vi "fpga_all_example2.vi"() -> ()   [LabVIEW 2020]
uses:
  controls/enum.ctl
  <vilib>/Platform/TimedLoop/XDataNode/timing_clust.ctl
  <vilib>/Platform/TimedLoop/XDataNode/nitl_modes.ctl
  <vilib>/Platform/TimedLoop/XDataNode/wakeup.ctl
  <vilib>/rvi/Emulation/niFpgaGetClockAttributes.vi
  <vilib>/rvi/Emulation/niFpgaSctlEmulationGetInTimedLoop.vi
  <vilib>/rvi/Emulation/niFpgaEmulationReportErrorSimple.vi
  <vilib>/rvi/Emulation/niFpgaCriticalErrorInLSC.vi
  <vilib>/rvi/Emulation/niFpgaProcessEmulError.vi
  <vilib>/rvi/eio/common/nirviEmuTemplateMethod_errors.vi
  lib/Cast-EPICS/cast u64 to u-64-64.vi
  lib/Cast-EPICS/cast u-64-64 to u64.vi
  lib/Cast-EPICS/cast u64 to u-64-0.vi
  lib/Cast-EPICS/cast u-64-0 to u64.vi
  lib/Cast-EPICS/cast u64 to u-64-32.vi
  lib/Cast-EPICS/cast u-64-32 to u64.vi
  lib/Cast-EPICS/cast u64 to s-64-0.vi
  lib/Cast-EPICS/cast s-64-0 to u64.vi
  lib/Cast-EPICS/cast u64 to s-64-64.vi
  lib/Cast-EPICS/cast s-64-64 to u64.vi
  lib/Cast-EPICS/cast u64 to s-64-32.vi
  lib/Cast-EPICS/cast s-64-32 to u64.vi
  <vilib>/Platform/TimedLoop/XDataNode/XDataNode.xnode
  <vilib>/eio/EIONode/EIONode.xnode
  <vilib>/Platform/TimedLoop/XDataNode/XDNodeRunTimeDep.lvlib
  lib/Scaler-EPICS/scaler.lvlib
  lib/Cast-EPICS/fixedpoint-cast.lvlib
panel:
  out "MBBI0":T1
  out "MBBI1":T1
  in  "MBBO1":T1
  in  "MBBO0":T1
  out "AI3":sgl format="%.2f"
  out "AI2":sgl format="%.2f"
  out "AI1":sgl format="%.2f"
  out "AI0":sgl format="%.2f"
  in  "AO3":sgl
  in  "AO2":sgl
  in  "AO1":sgl
  in  "AO0":sgl
  out "fixedpoint_i 1":fxp<+,64,64> format="%.20f"
  out "FXP1":u64
  out "fixedpoint_i 2":fxp<+,64,0> format="%#_20g"
  out "FXP2":u64
  out "fixedpoint_i 3":fxp<+,64,32> format="%#_20g"
  out "FXP3":u64
  out "fixedpoint_i 4":fxp<+/-,64,0> format="%#_20g"
  out "FXP4":u64
  out "fixedpoint_i 5":fxp<+/-,64,64> format="%.20f"
  out "FXP5":u64
  out "fixedpoint_i 6":fxp<+/-,64,32> format="%#_20g"
  out "FXP6":u64
  in  "FXP1":u64
  in  "FXP2":u64
  in  "FXP3":u64
  in  "FXP4":u64
  in  "FXP5":u64
  in  "FXP6":u64
  out "AnalogInputs_Scaler":fxp<+/-,20,5>[](array[numeric]) format="%.17g"
  out "Looptime":u32
  in  "Enable_SCALER":bool
  in  "OneShot_SCALER":bool
  in  "SampleAnalog_SCALER":bool
  in  "Gate_SCALER":bool[](array[boolean])=[FALSE, FALSE, FALSE, FALSE, FALSE]
  in  "PresetValues_SCALER":u32[](array[numeric])=[0, 0, 0, 0, 0]
  in  "fxp_ShiftLeft_SCALER":u64
  out "Done_SCALER":bool
  out "fxp_AnalogOutput0_SCALER":u64
  out "fxp_AnalogOutput1_SCALER":u64
  out "fxp_AnalogOutput2_SCALER":u64
  out "fxp_AnalogOutput3_SCALER":u64
  out "Counter_SCALER":u32[](array[numeric])
  out "BI_VECTOR":u64
  in  "BO3":bool
  out "BI_led3":bool
  out "BI_led2":bool
  in  "BO2":bool
  in  "BO1":bool
  out "BI_led1":bool
  out "BI_led0":bool
  in  "BO0":bool
  # "MBBI/MBBO Tests"
  # "BI/BO tests"
  # "AI/AO Tests"
  # "Scaler test"
  # "FXP test"
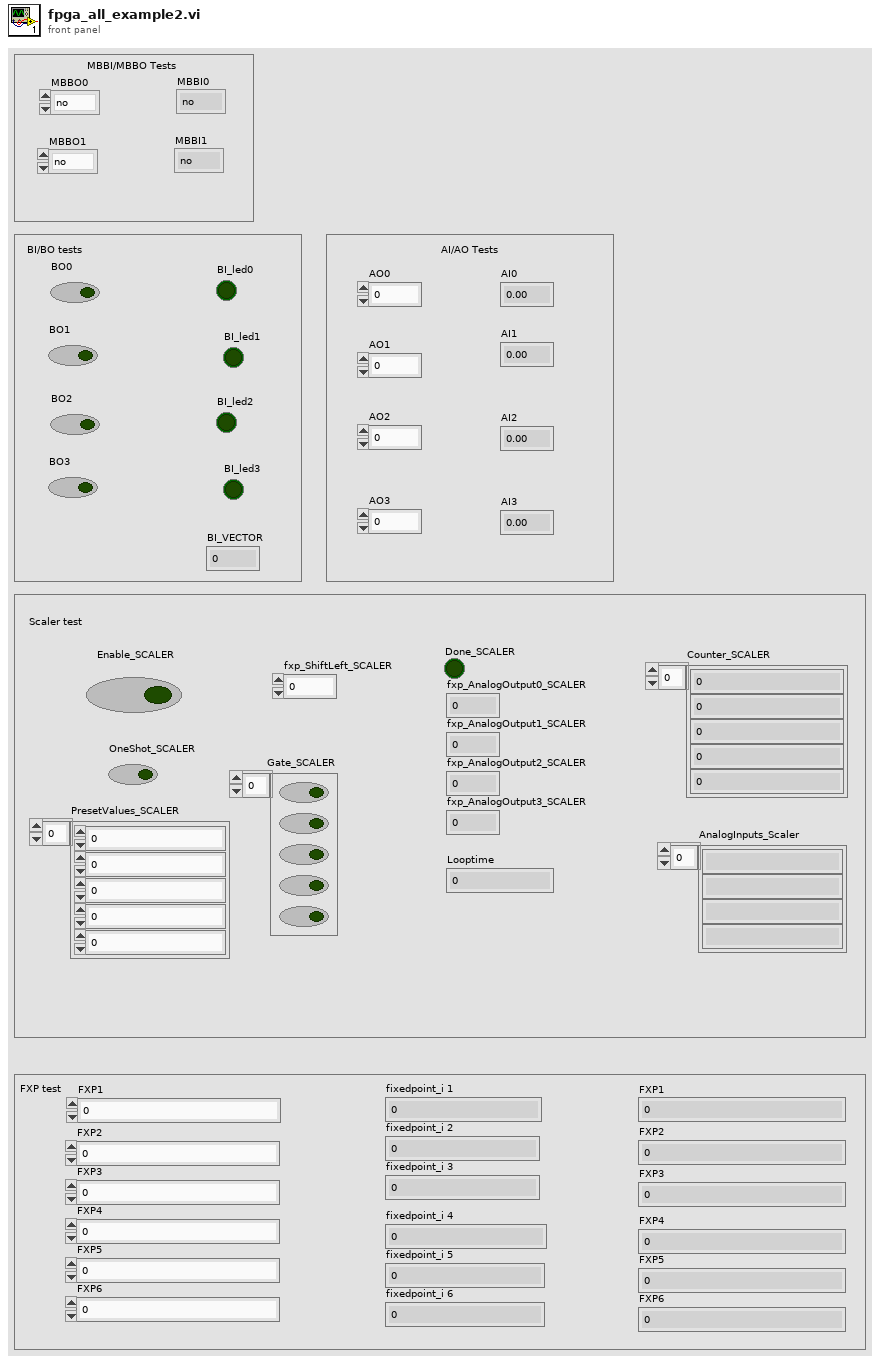
[diagram p1: front panel]
types:
  T1 = typedef "enum.ctl" = enum16{"no", "yes", "dont know"}
  T2 = typedef "XDNodeRunTimeDep.lvlib/timing_clust.ctl" = cluster{"Expected End [f-1]":u64, "Actual End [f-1]":u64, "Finished Late? [f-1]":bool, "Expected End [i-1]":u64, "Actual End [i-1]":u64, "Finished Late? [i-1]":bool, "Expected Start [i]":u64, "Actual Start [i]":u64, "Expected Start [f]":u64, "Actual Start [f]":u64, "Source Name":string, "Structure Name":string, "Period":i64, "Deadline":i64, "Offset":i64, "Start":i64, "Priority":i32, "Timeout":i32, "Mode":T3, "Wakeup Reason":T4, "Error":errorcluster, "Source Type":string, "Secondary Source Type":string, "Global End Time":u64, "Global Start Time":u64, "Frame Duration":u64, "Iteration Duration":u64, "Assigned CPU":i32, "I/O Scan Engine Mode":u32}
  T3 = typedef "XDNodeRunTimeDep.lvlib/nitl_modes.ctl" = enum32{"No Change", "Process missed periods, maintain original phase", "Discard missed periods, maintain original phase", "Process missed periods, ignore original phase", "Discard missed periods, ignore original phase"}
  T4 = typedef "XDNodeRunTimeDep.lvlib/wakeup.ctl" = enum32{"Normal", "Aborted", "Asynchronous wakeup", "Timing source error", "Timed loop error", "Timeout"}
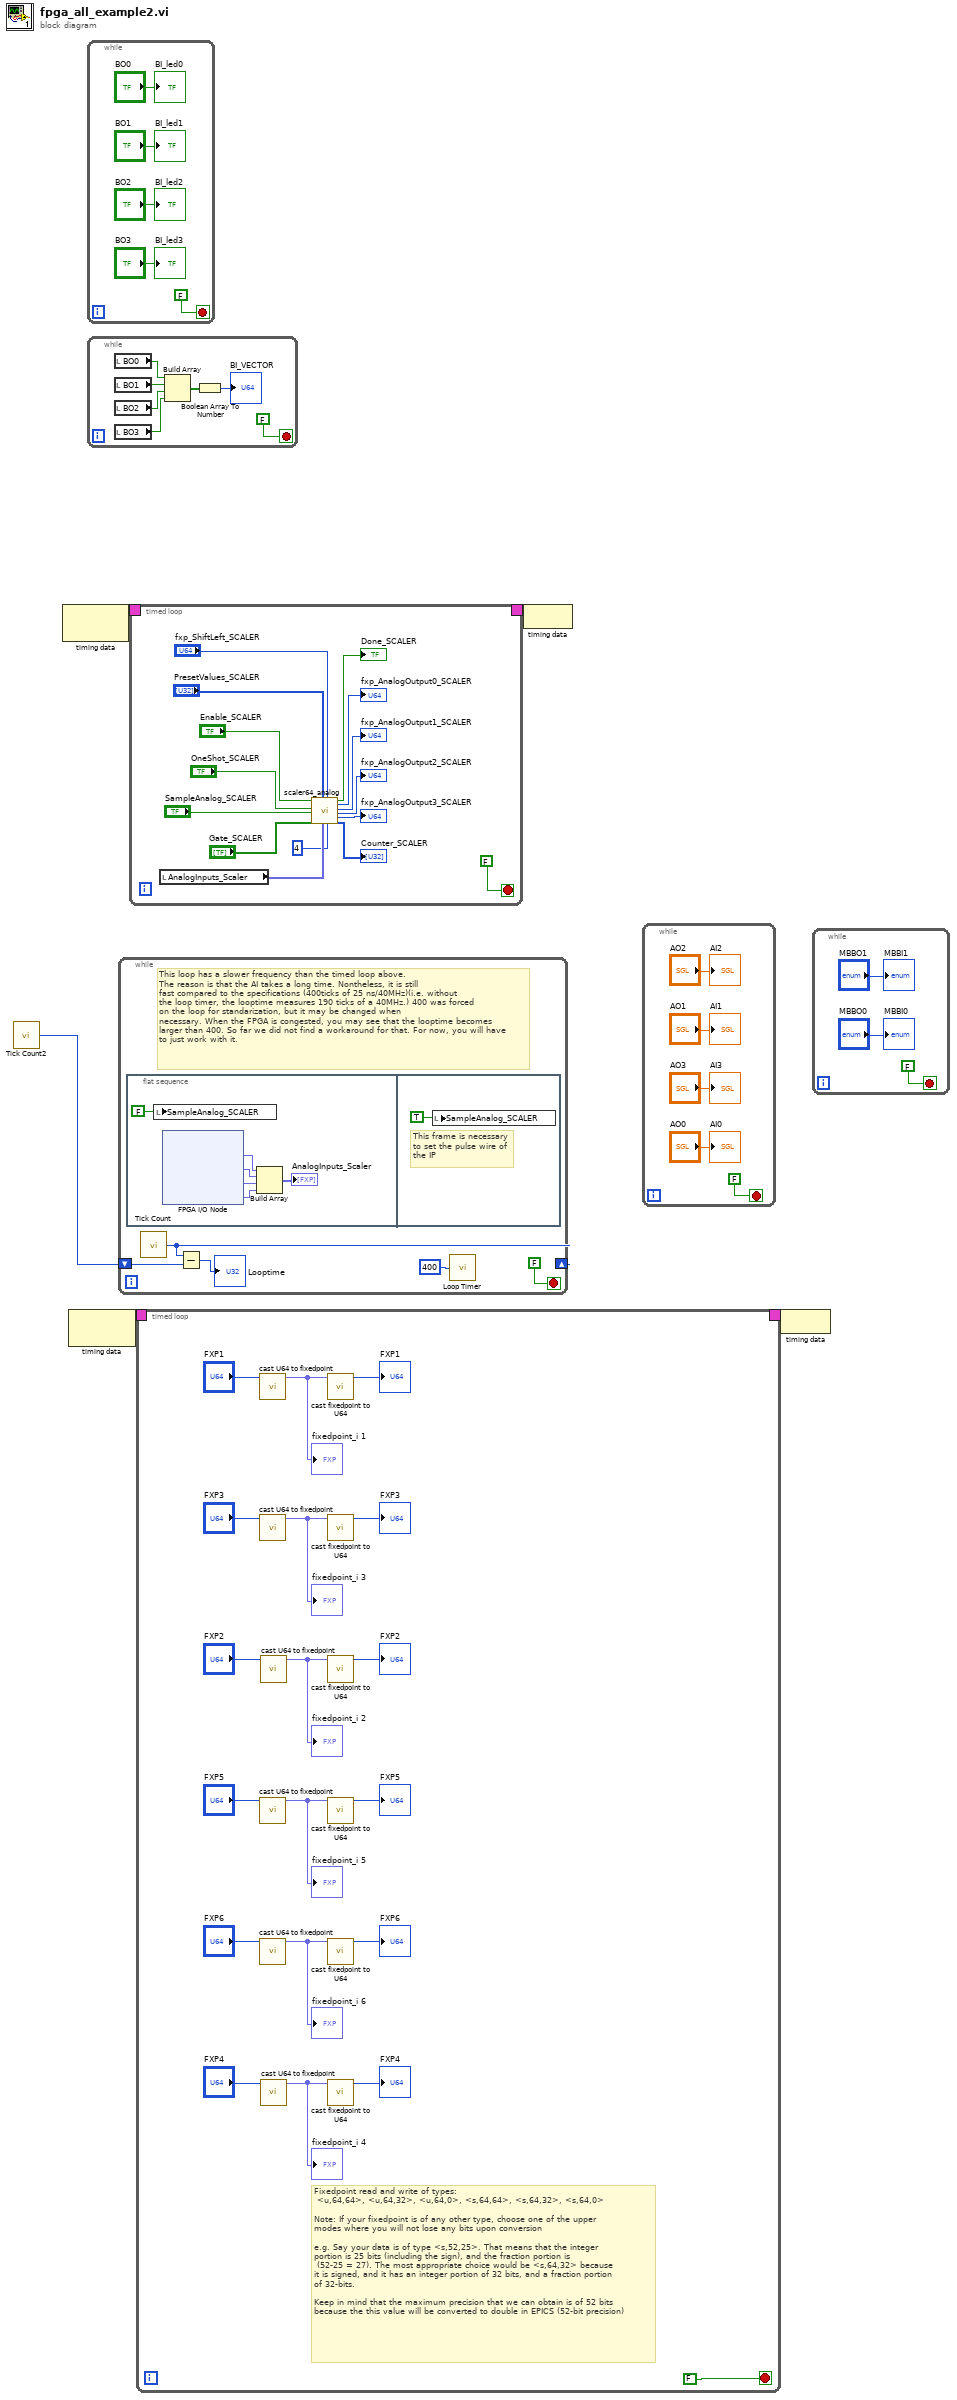
[diagram p0: block diagram]
diagram:
  n1 = call "Tick Count2"() -> ("Tick Count(Ticks)"=w3:u32)
  n2 = node-c288() -> (w5:T2)  [unwired: 1 in]
  n3 = node-c288() -> (w2:T2)  [unwired: 1 in]
  n4 = while {
    stop <- FALSE stop-if-true
    "BI_led0" <- "BO0"
    "BI_led1" <- "BO1"
    "BI_led2" <- "BO2"
    "BI_led3" <- "BO3"
  }
  n5 = while {
    stop <- FALSE stop-if-true
    n6 = local read "BO0"() -> (w14:bool)
    n7 = local read "BO1"() -> (w12:bool)
    n8 = local read "BO2"() -> (w13:bool)
    n9 = local read "BO3"() -> (w15:bool)
    n10 = Build Array(w14, w12, w13, w15) -> (w16:bool[])
    n11 = Boolean Array To Number(Boolean array=w16) -> (number=→"BI_VECTOR":u8)
  }
  n12 = while {
    shift-right: [w19] -> _
    shift-left: w3 -> [w20]
    stop <- FALSE stop-if-true
    # "This loop has a slower frequency than the timed loop above.\nThe reason is that the AI takes a long time. Nontheless, it is still\nfast compared to the specifications (400ticks of 25 ns/40MHz)(i.e. without \nthe loop timer, the looptime measures 190 ticks of a 40MHz.) 400 was forced \non the loop for standarization, but it may be changed when \nnecessary. When the FPGA is congested, you may see that the looptime becomes \nlarger than 400. So far we did not find a workaround for that. For now, you will have\nto just work with it."
    n13 = flat-sequence {
      frame #0 {
        n14 = local write "SampleAnalog_SCALER"(FALSE) -> ()
        n15 = xnode "FPGA I/O Node"() -> ("Mod4/AI0"=w28:fxp<+/-,20,5>, "Mod4/AI1"=w26:fxp<+/-,20,5>, "Mod4/AI2"=w25:fxp<+/-,20,5>, "Mod4/AI3"=w24:fxp<+/-,20,5>)  [unwired: 4 in, 4 out]
        n16 = Build Array(w28, w26, w25, w24) -> (→"AnalogInputs_Scaler":fxp<+/-,20,5>[])
      }
      frame #1 {
        # "This frame is necessary to set the pulse wire of the IP"
        n17 = local write "SampleAnalog_SCALER"(TRUE ("sample")) -> ()
      }
    }
    n18 = call "Tick Count"() -> ("Tick Count(Ticks)"=w19:u32)
    n19 = Subtract(x=w19, y=w20) -> (x-y=→"Looptime":u32)
    n20 = call "Loop Timer"("Count(Ticks)"=i16 400) -> ()  [unwired: 1 out]
  }
  n21 = timed-loop {
    timing: w5 -> [_]
    timing-out: [_] -> w4
    stop <- FALSE stop-if-true
    n22 = local read "AnalogInputs_Scaler"() -> (w43:fxp<+/-,20,5>[])
    n23 = call "scaler64_analog.vi"("Enable_SCALER"="Enable_SCALER", "OneShot_SCALER"="OneShot_SCALER", "SampleAnalog_SCALER"="SampleAnalog_SCALER", "Gate_SCALER"="Gate_SCALER", "PresetValues_SCALER"="PresetValues_SCALER", "AnalogInputs_SCALER"=w43, "fxp_ShiftLeft_SCALER"="fxp_ShiftLeft_SCALER", "divisor_SCALER"=i16 4) -> ("Done_SCALER"=→"Done_SCALER":bool, "fxp_RawAI0_SCALER"=→"fxp_AnalogOutput0_SCALER":u64, "fxp_RawAI1_SCALER"=→"fxp_AnalogOutput1_SCALER":u64, "fxp_RawAI2_SCALER"=→"fxp_AnalogOutput2_SCALER":u64, "fxp_RawAI3_SCALER"=→"fxp_AnalogOutput3_SCALER":u64, "Counter_SCALER"=→"Counter_SCALER":u32[])  [unwired: 5 in, 1 out]
  }
  n24 = timed-loop {
    timing: w2 -> [_]
    timing-out: [_] -> w1
    stop <- FALSE stop-if-true
    # "Fixedpoint read and write of types:\n <u,64,64>, <u,64,32>, <u,64,0>, <s,64,64>, <s,64,32>, <s,64,0>\n\nNote: If your fixedpoint is of any other type, choose one of the upper\nmodes where you will not lose any bits upon conversion\n\ne.g. Say your data is of type <s,52,25>. That means that the integer\nportion is 25 bits (including the sign), and the fraction portion is\n (52-25 = 27). The most appropriate choice would be <s,64,32> because\nit is signed, and it has an integer portion of 32 bits, and a fraction portion\nof 32-bits. \n\nKeep in mind that the maximum precision that we can obtain is of 52 bits\nbecause the this value will be converted to double in EPICS (52-bit precision)"
    n25 = call-poly "cast U64 to fixedpoint.vi"("aofxp"="FXP1") -> ("fixedpoint_o"=w58:fxp<+,64,64>)  [unwired: 10 in]
    "fixedpoint_i 1" <- w58
    n26 = call-poly "cast U64 to fixedpoint.vi"("aofxp"="FXP3") -> ("fixedpoint_o"=w53:fxp<+,64,32>)  [unwired: 10 in]
    "fixedpoint_i 3" <- w53
    n27 = call-poly "cast U64 to fixedpoint.vi"("aofxp"="FXP5") -> ("fixedpoint_o"=w55:fxp<+/-,64,64>)  [unwired: 10 in]
    "fixedpoint_i 5" <- w55
    n28 = call-poly "cast U64 to fixedpoint.vi"("aofxp"="FXP6") -> ("fixedpoint_o"=w56:fxp<+/-,64,32>)  [unwired: 10 in]
    "fixedpoint_i 6" <- w56
    n29 = call-poly "cast U64 to fixedpoint.vi"("aofxp"="FXP2") -> ("fixedpoint_o"=w54:fxp<+,64,0>)  [unwired: 10 in]
    "fixedpoint_i 2" <- w54
    n30 = call-poly "cast U64 to fixedpoint.vi"("aofxp"="FXP4") -> ("fixedpoint_o"=w57:fxp<+/-,64,0>)  [unwired: 10 in]
    "fixedpoint_i 4" <- w57
    n31 = call-poly "cast fixedpoint to U64.vi"("fixedpoint_i"=w58) -> ("aifxp"=→"FXP1":u64)  [unwired: 10 in]
    n32 = call-poly "cast fixedpoint to U64.vi"("fixedpoint_i"=w53) -> ("aifxp"=→"FXP3":u64)  [unwired: 10 in]
    n33 = call-poly "cast fixedpoint to U64.vi"("fixedpoint_i"=w54) -> ("aifxp"=→"FXP2":u64)  [unwired: 10 in]
    n34 = call-poly "cast fixedpoint to U64.vi"("fixedpoint_i"=w55) -> ("aifxp"=→"FXP5":u64)  [unwired: 10 in]
    n35 = call-poly "cast fixedpoint to U64.vi"("fixedpoint_i"=w56) -> ("aifxp"=→"FXP6":u64)  [unwired: 10 in]
    n36 = call-poly "cast fixedpoint to U64.vi"("fixedpoint_i"=w57) -> ("aifxp"=→"FXP4":u64)  [unwired: 10 in]
  }
  n37 = node-c288(w4) -> ()
  n38 = while {
    stop <- FALSE stop-if-true
    "AI0" <- "AO0"
    "AI1" <- "AO1"
    "AI2" <- "AO2"
    "AI3" <- "AO3"
  }
  n39 = node-c288(w1) -> ()
  n40 = while {
    stop <- FALSE stop-if-true
    "MBBI0" <- "MBBO0"
    "MBBI1" <- "MBBO1"
  }
